vi "By Value Behaviour.vi"() -> ()   [LabVIEW 2010]
uses:
  <vilib>/MDSplus/Classes/Tree_Class/Tree.lvclass
  <vilib>/MDSplus/Classes/Data_Class/TreeNode_Class/TreeNode.lvclass
  <vilib>/MDSplus/Classes/Data_Class/Data.lvclass
  <vilib>/MDSplus/Classes/Data_Class/Scalar_Class/Float32_Class/Float32.lvclass
panel:
  out "SGL out 2":sgl
  in  "SGL in":sgl=5.555
  out "SGL out":sgl
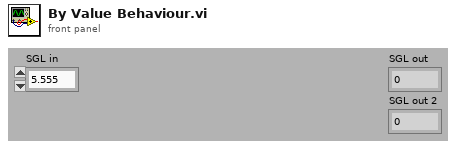
[diagram p1: front panel]
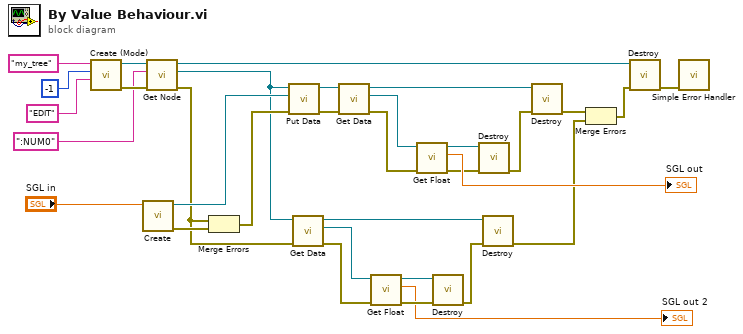
[diagram p0: block diagram]
diagram:
  n1 = call <vilib>:"Create (Mode).vi"("Mode"="EDIT", "Shot"=-1, "Name"="my_tree") -> ("error out"=w29:errorcluster, "Tree out"=w33:refnum<class "Tree.lvclass">)  [unwired: 7 in]
  n2 = call <vilib>:"Create.vi"("SGL in"="SGL in") -> ("error out"=w23:errorcluster, "Float32 out"=w26:refnum<class "Float32.lvclass">)  [unwired: 9 in]
  n3 = call-dynamic "Get Node.vi"("error in (no error)"=w29, "Path"=":NUM0", "Tree in"=w33) -> ("error out"=w7:errorcluster, "Node out"=w8:refnum<class "TreeNode.lvclass">, "Tree out"=w25:refnum<class "Tree.lvclass">)  [unwired: 6 in]
  n4 = Merge Errors(w7, w23) -> (w24:errorcluster)
  n5 = call-dynamic "Put Data.vi"("error in (no error)"=w24, "Data"=w26, "TreeNode in"=w8) -> ("error out"=w21:errorcluster, "TreeNode out"=w22:refnum<class "TreeNode.lvclass">)  [unwired: 7 in]
  n6 = call-dynamic "Get Data.vi"("error in (no error)"=w7, "TreeNode in"=w8) -> ("error out"=w10:errorcluster, "Data out"=w9:refnum<class "Data.lvclass">, "TreeNode out"=w5:refnum<class "TreeNode.lvclass">)  [unwired: 7 in]
  n7 = call-dynamic "Get Data.vi"("error in (no error)"=w21, "TreeNode in"=w22) -> ("error out"=w18:errorcluster, "Data out"=w19:refnum<class "Data.lvclass">, "TreeNode out"=w20:refnum<class "TreeNode.lvclass">)  [unwired: 7 in]
  n8 = call-dynamic "Get Float.vi"("error in (no error)"=w10, "Data in"=w9) -> ("error out"=w12:errorcluster, "SGL out"=→"SGL out 2":sgl, "Data out"=w11:refnum<class "Data.lvclass">)  [unwired: 7 in]
  n9 = call-dynamic "Get Float.vi"("error in (no error)"=w18, "Data in"=w19) -> ("error out"=w15:errorcluster, "SGL out"=→"SGL out":sgl, "Data out"=w17:refnum<class "Data.lvclass">)  [unwired: 7 in]
  n10 = call-dynamic "Destroy.vi"("error in (no error)"=w12, "Data in"=w11) -> ("error out"=w4:errorcluster)  [unwired: 9 in]
  n11 = call-dynamic "Destroy.vi"("error in (no error)"=w15, "Data in"=w17) -> ("error out"=w14:errorcluster)  [unwired: 9 in]
  n12 = call-dynamic "Destroy.vi"("error in (no error)"=w4, "TreeNode in"=w5) -> ("error out"=w2:errorcluster)  [unwired: 9 in]
  n13 = call-dynamic "Destroy.vi"("error in (no error)"=w14, "TreeNode in"=w20) -> ("error out"=w3:errorcluster)  [unwired: 9 in]
  n14 = Merge Errors(w3, w2) -> (w1:errorcluster)
  n15 = call-dynamic "Destroy.vi"("error in (no error)"=w1, "Tree in"=w25) -> ("error out"=w13:errorcluster)  [unwired: 9 in]
  n16 = call <vilib>:"Simple Error Handler.vi"("error in (no error)"=w13) -> ()  [unwired: 4 in, 5 out]
